vi "main 2.18.22.vi"() -> ()   [LabVIEW 2021]
uses:
  <vilib>/express/express arith-compare/Formula/XNode/ExpressFormulaBlockNode.xnode
  <vilib>/ptbypt/NI_PtbyPt.lvlib
panel:
  out "Waveform Chart 4":waveform(dbl)(graph)
  out "Thermistor Filtered":dbl[](graph)
  out "Thermistor Unfiltered":dbl[](graph)
  in  "Thermistor":T1
  out "Waveform Chart 3":T2(graph)
  in  "error in (no error)":errorcluster
  out "error out":errorcluster
  out "Waveform Chart 2":waveform(dbl)(graph)
  out "a0 Scalar":dbl
  out "Waveform Chart":dynamicdata(graph)
  in  "stop":bool
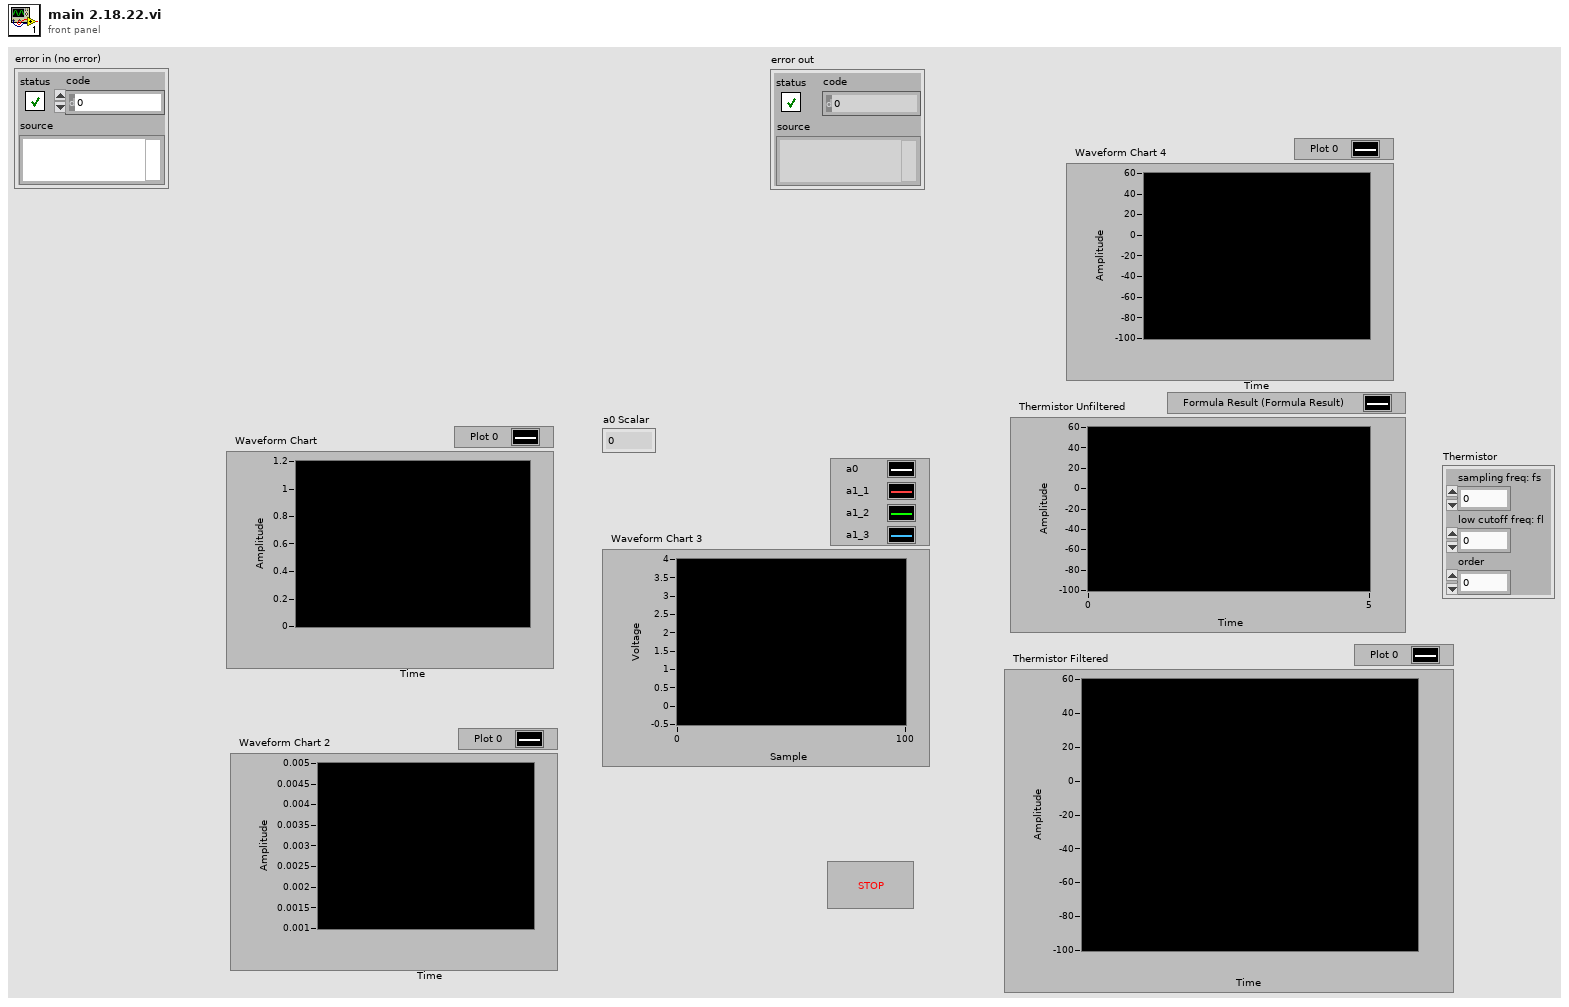
[diagram p1: front panel]
types:
  T1 = cluster{"sampling freq: fs":dbl, "low cutoff freq: fl":dbl, "order":i32}
  T2 = cluster{"Data_Array[0]":dbl, "Data_Array[1]":dbl, "Data_Array[2]":dbl, "Data_Array[3]":dbl, "Data_Array[4]":dbl, "Data_Array[5]":dbl, "Data_Array[6]":dbl, "Data_Array[7]":dbl, "Data_Array[8]":dbl}
  T3 = cluster{"Data_Array":dbl[], "Multiplex_Tbl":u32[]}
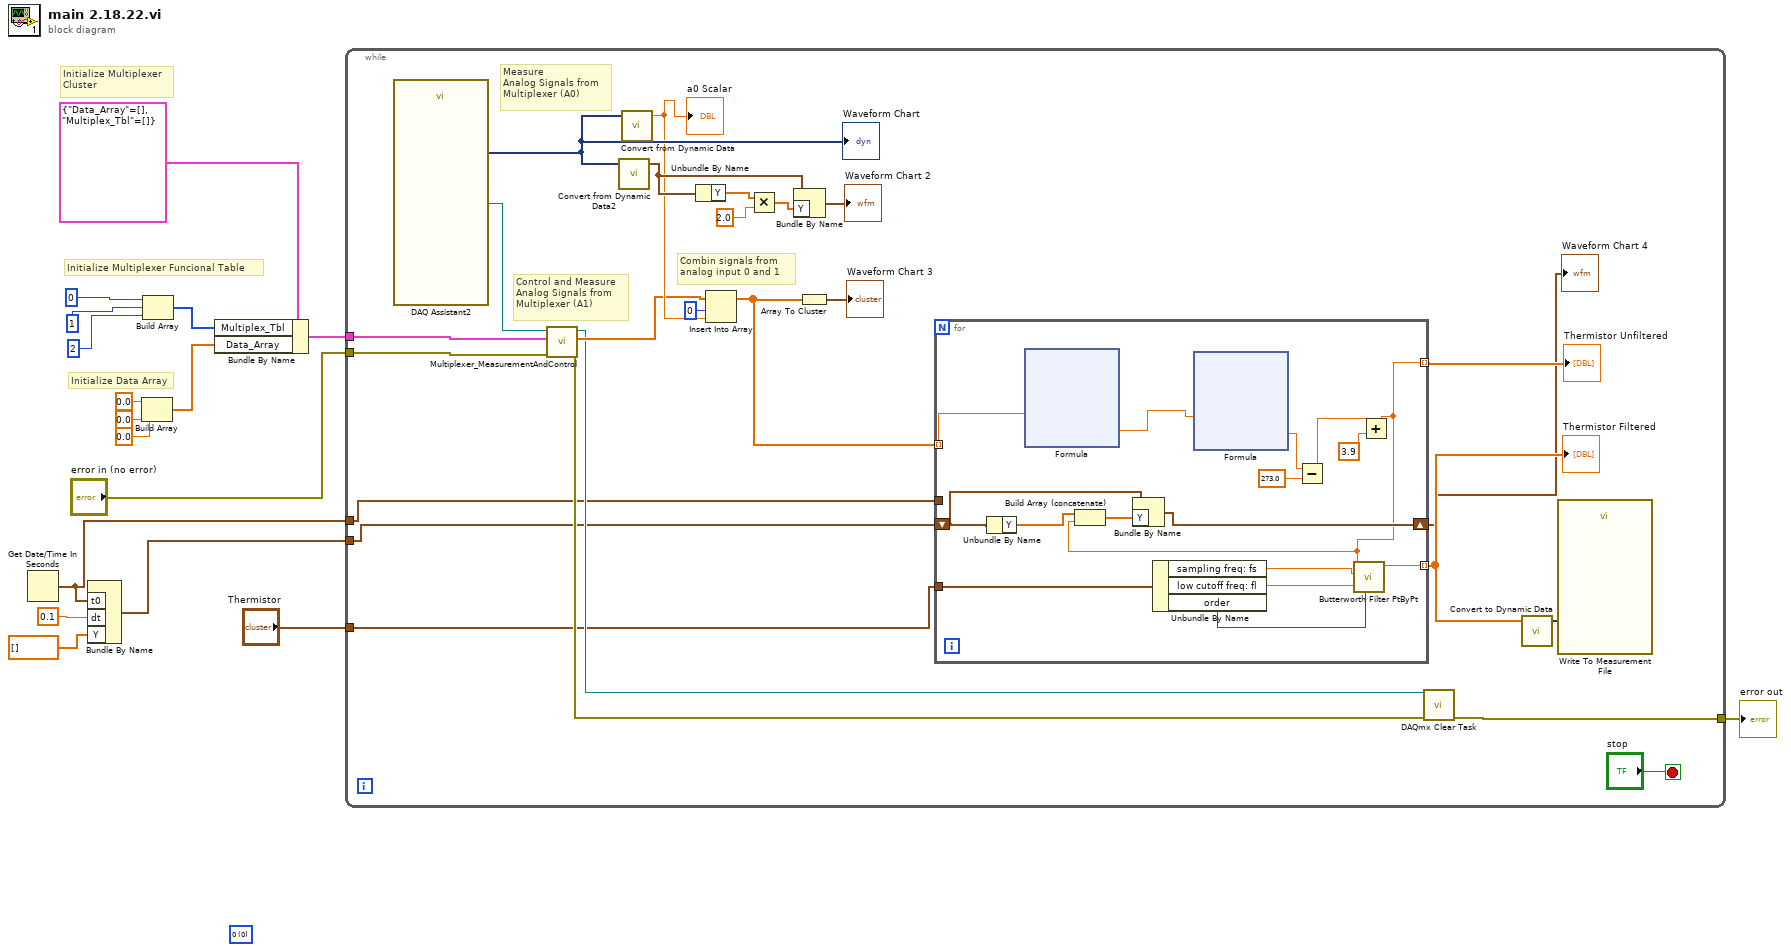
[diagram p0: block diagram]
diagram:
  (unwired) u8 0 items=["0", "1", "Z", "L", "H", "X", "T", "V"] ("digital values ring")
  # "Initialize Multiplexer \nCluster"
  # "Initialize Data Array"
  # "Initialize Multiplexer Funcional Table"
  n1 = Get Date/Time In Seconds() -> (seconds since 1Jan1904=w1:timestamp)
  n2 = Bundle By Name("t0"=w1, "dt"=0.1, "Y"=dbl[] []) -> (w2:waveform(dbl))  [unwired: 1 in]
  n3 = Build Array(0.0 ("element"), 0.0 ("element"), 0.0 ("element")) -> (w13:dbl[])
  n4 = Build Array(u32 0 ("Waveform"), 1 ("Waveform"), u32 2 ("Waveform")) -> (w7:u32[])
  n5 = Bundle By Name(cluster=T3 {"Data_Array"=[], "Multiplex_Tbl"=[]}, "Multiplex_Tbl"=w7, "Data_Array"=w13) -> (w12:T3)
  n6 = while {
    tunnel: w12 -> [w35]
    tunnel: "error in (no error)" -> [w34]
    tunnel: [w26] -> w6
    tunnel: "Thermistor" -> [w25]
    tunnel: w2 -> [w20]
    tunnel: w1 -> [w18]
    stop <- "stop" stop-if-true
    # "Combin signals from \nanalog input 0 and 1"
    # "Measure\nAnalog Signals from\nMultiplexer (A0)"
    # "Control and Measure\nAnalog Signals from\nMultiplexer (A1)"
    n7 = call "DAQ Assistant2"() -> ("task out"=w33:refnum<k21>, "data"=w36:dynamicdata)  [unwired: 16 in, 2 out]
    "Waveform Chart" <- w36
    n8 = call "Multiplexer_MeasurementAndControl.vi"("error in (no error)"=w34, "Multiplexer_Cluser"=w35, "Task in"=w33) -> ("error out"=w27:errorcluster, "Data_Array"=w30:dbl[], "Task out"=w28:refnum<k21>)  [unwired: 6 in]
    n9 = call "Convert from Dynamic Data2"("Dynamic Data Type"=w36) -> ("Waveform"=w39:waveform(dbl))  [unwired: 3 in]
    n10 = call "Convert from Dynamic Data"("Dynamic Data Type"=w36) -> ("Scalar"=w32:dbl)  [unwired: 3 in]
    "a0 Scalar" <- w32
    n11 = Unbundle By Name(w39) -> ("Y"=w41:dbl[])
    n12 = Insert Into Array(array=w30, index=0, new element=w32) -> (w24:dbl[])
    n13 = Multiply(x=w41, y=2.0) -> (x*y=w38:dbl[])
    n14 = Bundle By Name(cluster=w39, "Y"=w38) -> (→"Waveform Chart 2":waveform(dbl))
    n15 = Array To Cluster(array=w24) -> (cluster=→"Waveform Chart 3":T2)
    n16 = for {
      tunnel: w24 -> [w50] mode=indexing
      tunnel: w25 -> [w49]
      tunnel: [w46] -> w22 mode=indexing
      tunnel: [w48] -> w21 mode=indexing
      tunnel: w18 -> [_]
      shift-right: [w47] -> w19
      shift-left: w20 -> [w44]
      n17 = Unbundle By Name(w44) -> ("Y"=w43:dbl[])
      n18 = xnode "Formula"("v"=w50) -> ("Result"=w57:dbl)  [unwired: 1 in, 1 out]
      n19 = Unbundle By Name(w49) -> ("sampling freq: fs"=w56:dbl, "low cutoff freq: fl"=w55:dbl, "order"=w54:i32)
      n20 = xnode "Formula"("R"=w57) -> ("Result"=w52:dbl)  [unwired: 1 in, 1 out]
      n21 = Subtract(x=w52, y=273.0) -> (x-y=w51:dbl)
      n22 = Add(x=w51, y=3.9) -> (x+y=w46:dbl)
      n23 = Build Array (concatenate)(w43, w46) -> (w45:dbl[])
      n24 = Bundle By Name(cluster=w44, "Y"=w45) -> (w47:waveform(dbl))
      n25 = call <vilib>:"Butterworth Filter PtByPt.vi"("order"=w54, "low cutoff freq: fl"=w55, "sampling freq: fs"=w56, "x"=w46) -> ("Filtered x"=w48:dbl)  [unwired: 5 in, 1 out]
    }
    "Thermistor Unfiltered" <- w22
    "Thermistor Filtered" <- w21
    "Waveform Chart 4" <- w19
    n26 = call <vilib>:"DAQmx Clear Task.vi"("task in"=w28, "error in"=w27) -> ("error out"=w26:errorcluster)  [unwired: 13 in]
    n27 = call "Convert to Dynamic Data"("Array"=w21) -> ("Dynamic Data Type"=w23:dynamicdata)  [unwired: 3 in]
    n28 = call "Write To Measurement File"("Signals"=w23) -> ()  [unwired: 16 in, 3 out]
  }
  "error out" <- w6
